vi "2012_12_14_local.vi"(0 "MC Power Data In":waveform(dbl)[](array[waveform]), 1 "Motor Power Data In":waveform(dbl)[](array[waveform]), 5 "Power \nSetting":i8(slide) min=0 max=100 step=10 scale=0.0..100.0, 7 "On/Off Control":T1(ring), 9 "Motor":i16=1, 11 "Error In":errorcluster, 12 "Fine Data In":dbl[][][](array[numeric])) -> (6 "Power \nSetting":i8(slide) min=0 max=100 step=10 scale=0.0..100.0, 14 "Fine Data Out":dbl[][][](array[numeric]), 15 "Errors":errorcluster)   [LabVIEW 2011]
uses:
  <vilib>/express/express arith-compare/Formula/XNode/ExpressFormulaBlockNode.xnode
  <vilib>/Analysis/NI_AALBase.lvlib
panel:
  in  "coarse path":path=path "Durability/coarse.lvm"
  in  "fine path":path=path "Durability/fine.lvm"
  out "Efficiency (%)":dbl format="%#.4f"
  in  "Manual Save\nFine Event":bool
  in  "Motor1 ID":string
  in  "User":string
  in  "Comments (cleared when written to file)":string
  out "Elapsed Time (s)":string caption="Elapsed Time Text"
  out "Start Time":string caption="Start Time Text"
  in  "Motor Failure\n(click to reset)":bool
  out "Coarse":bool caption="Time has Elapsed"
  out "Fine":bool caption="Time has Elapsed"
  out "Temps":dynamicdata(graph) caption="Signal Out"
  out "Power Graph":dynamicdata(graph) caption="Collected Signals"
  out "RPM":dynamicdata(graph) caption="Collected Signals"
  out "Motor RPM":dbl format="%#.0f"
  out "Power to Motor (W)":dbl format="%#.4f"
  out "Power to MC (W)":dbl format="%#.4f"
  out "Supply Voltage (V)":dbl format="%#.4f"
  in  "Record":bool
  out "Motor Temp (F)":dbl format="%.1f"
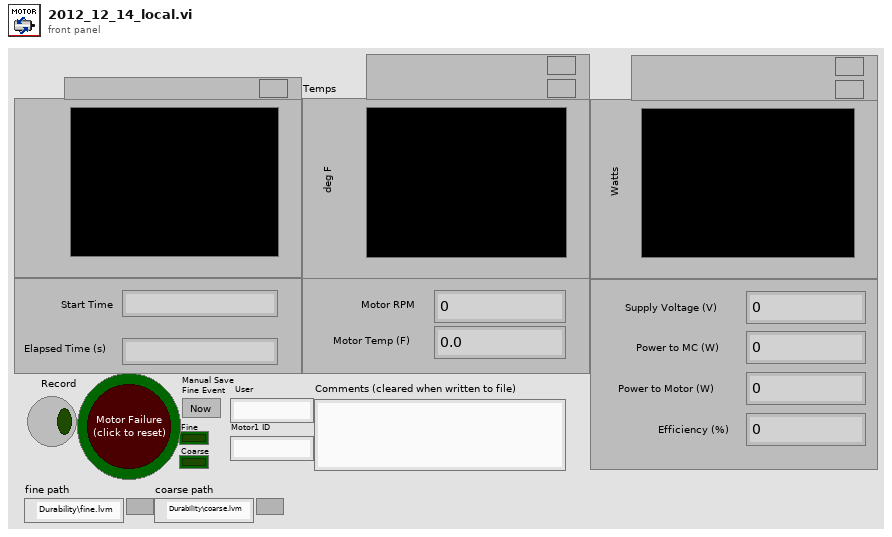
[diagram p1: front panel]
types:
  T1 = enum8{"Enabled", "Disabled", "Disabled and Grayed Out"}
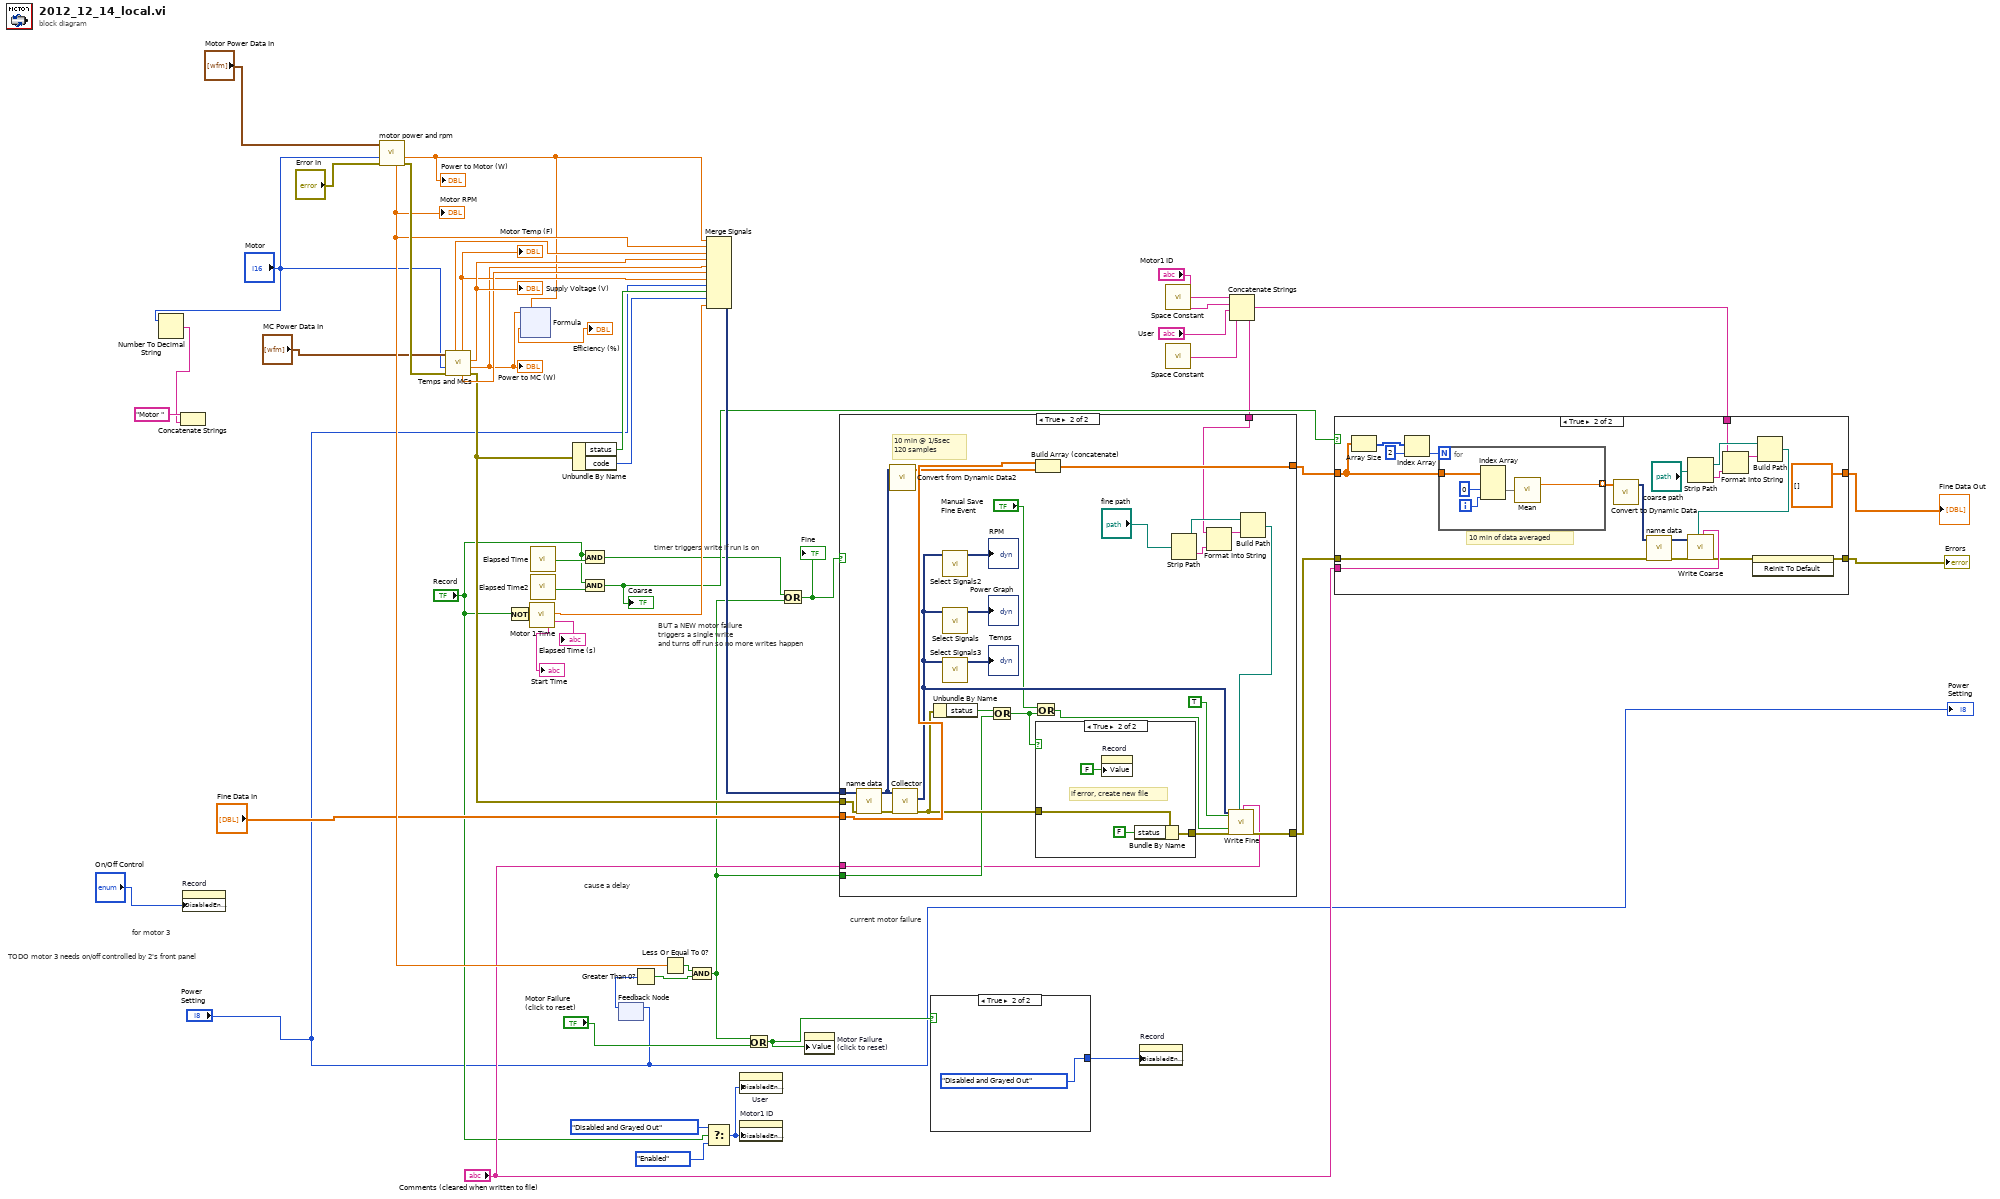
[diagram p0: block diagram]
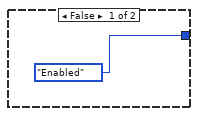
[diagram p2: hidden frame]
diagram:
  # "TODO motor 3 needs on/off controlled by 2's front panel"
  # "for motor 3"
  # "cause a delay"
  # "timer triggers write if run is on"
  # "BUT a NEW motor failure\ntriggers a single write\nand turns off run so no more writes happen"
  # "current motor failure"
  n1 = Number To Decimal String(number="Motor") -> (decimal integer string=w14:string)  [unwired: 1 in]
  n2 = Concatenate Strings("Motor ", w14) -> ()  [unwired: 1 out]
  n3 = property on="Record" class="Bool (strict)"("DisabledEnum"="On/Off Control") -> ()  [unwired: 2 in, 2 out]
  n4 = call "motor power and rpm.vi"("error in (no error)"="Error In", "Motor"="Motor", "data"="Motor Power Data In") -> ("error out"=w52:errorcluster, "Power"=w29:dbl, "RPM"=w42:dbl)  [unwired: 4 in, 2 out]
  "Motor RPM" <- w42
  "Power to Motor (W)" <- w29
  n5 = call "Temps and MCs.vi"("error in (no error)"=w52, "Motor"="Motor", "data"="MC Power Data In") -> ("error out"=w17:errorcluster, "Power 1"=w28:dbl, "Voltage 1"=w47:dbl, "Tank Temp"=w46:dbl, "Motor Temp"=w45:dbl, "Current 1"=w51:dbl)  [unwired: 3 in]
  "Motor Temp (F)" <- w45
  "Supply Voltage (V)" <- w47
  "Power to MC (W)" <- w28
  n6 = Not(x="Record") -> (.not. x?=w37:bool)
  n7 = xnode ("Formula")("MC PWR"=w28, "M PWR"=w29) -> ("Result"=→"Efficiency (%)":dbl)  [unwired: 1 in, 1 out]
  n8 = call "Motor 1 Time"("Reset"=w37) -> ("Start Time Text"=→"Start Time":string, "Elapsed Time (s)"=w36:dbl, "Elapsed Time Text"=→"Elapsed Time (s)":string)  [unwired: 11 in, 5 out]
  n9 = call "Elapsed Time"() -> ("Time has Elapsed"=w30:bool)  [unwired: 12 in, 7 out]
  n10 = call "Elapsed Time2"() -> ("Time has Elapsed"=w32:bool)  [unwired: 12 in, 7 out]
  n11 = Unbundle By Name(w17) -> ("status"=w50:bool, "code"=w49:i32)
  n12 = And(x="Record", y=w30) -> (x .and. y?=w5:bool)
  n13 = And(x="Record", y=w32) -> (x .and. y?=w31:bool)
  "Coarse" <- w31
  n14 = feedback-in #1("Power \nSetting") -> ()
  n15 = feedback #1() -> (w6:i8)  [unwired: 1 in]
  n16 = Greater Than 0?(x=w6) -> (x > 0?=w40:bool)
  n17 = Less Or Equal To 0?(x=w42) -> (x <= 0?=w41:bool)
  n18 = And(x=w41, y=w40) -> (x .and. y?=w4:bool)
  n19 = Merge Signals(w29, w42, w51, w47, w28, w46, w45, "Power \nSetting", w50, w49, w36) -> (w48:dynamicdata)
  n20 = Select(t=T1."Disabled and Grayed Out" ("Disabled"), s="Record", f=T1."Enabled" ("Disabled")) -> (s? t:f=w33:T1)
  n21 = property on="User" class="Str"("DisabledEnum"=w33) -> ()  [unwired: 2 in, 2 out]
  n22 = property on="Motor1 ID" class="Str"("DisabledEnum"=w33) -> ()  [unwired: 2 in, 2 out]
  n23 = Or(x=w4, y="Motor Failure\n(click to reset)") -> (x .or. y?=w2:bool)
  n24 = Or(x=w5, y=w4) -> (x .or. y?=w7:bool)
  "Fine" <- w7
  n25 = property on="Motor Failure\n(click to reset)" class="Bool (strict)"("Value"=w2) -> ()  [unwired: 2 in, 2 out]
  n26 = case shown="True" w2 {
    tunnel: [T1."Enabled" ("Disabled") T1."Disabled and Grayed Out" ("Disabled")] -> w9
    frame False {
    }
    frame True {
    }
  }
  n27 = property on="Record" class="Bool (strict)"("DisabledEnum"=w9) -> ()  [unwired: 2 in, 2 out]
  n28 = call <vilib>:"Space Constant.vi"() -> ("String"=w23:string)
  n29 = call <vilib>:"Space Constant.vi"() -> ("String"=w21:string)
  n30 = Concatenate Strings("Motor1 ID", w23, "User", w21) -> (w20:string)
  n31 = case shown="True" w7 {
    tunnel: w48 -> [_ w79]
    tunnel: w17 -> [w56 w76]
    tunnel: [w56 w71] -> w8
    tunnel: [w55 w83] -> w43
    tunnel: "Fine Data In" -> [w55 w82]
    tunnel: w4 -> [_ w68]
    tunnel: "Comments (cleared when written to file)" -> [_ w67]
    tunnel: w20 -> [_ w60]
    frame False {
    }
    frame True {
      # "10 min @ 1/5sec\n120 samples"
      n32 = call "name data.vi"("error in (no error)"=w76, "Dynamic Data"=w79) -> ("error out"=w77:errorcluster, "Output"=w78:dynamicdata)  [unwired: 8 in]
      n33 = call "Convert from Dynamic Data2"("Dynamic Data Type"=w78) -> ("Array"=w81:dbl[][])  [unwired: 3 in]
      n34 = call "Collector"("error in (no error)"=w77, "Signals"=w78) -> ("error out"=w69:errorcluster, "Collected Signals"=w72:dynamicdata)  [unwired: 8 in]
      n35 = Unbundle By Name(w69) -> ("status"=w58:bool)
      n36 = call "Select Signals2"("Signals"=w72) -> ("Signal Out"=→"RPM":dynamicdata)  [unwired: 9 in, 1 out]
      n37 = call "Select Signals"("Signals"=w72) -> ("Signal Out"=→"Power Graph":dynamicdata)  [unwired: 9 in, 1 out]
      n38 = call "Select Signals3"("Signals"=w72) -> ("Signal Out"=→"Temps":dynamicdata)  [unwired: 9 in, 1 out]
      n39 = Or(x=w58, y=w68) -> (x .or. y?=w57:bool)
      n40 = Or(x="Manual Save\nFine Event", y=w57) -> (x .or. y?=w66:bool)
      n41 = Build Array (concatenate)(w82, w81) -> (w83:dbl[][][])
      n42 = case shown="True" w57 {
        tunnel: [w84 w88] -> w70
        tunnel: w69 -> [w84 w87]
        frame False {
        }
        frame True {
          # "if error, create new file"
          n43 = property on="Record" class="Bool (strict)"("Value"=FALSE ("Manual Start")) -> ()  [unwired: 2 in, 2 out]
          n44 = Bundle By Name(cluster=w87, "status"=FALSE) -> (w88:errorcluster)
        }
      }
      n45 = Strip Path(path="fine path") -> (stripped path=w63:path, name=w59:string)
      n46 = Format Into String(initial string=w60, w59) -> (resulting string=w64:string)  [unwired: 2 in, 1 out]
      n47 = Build Path(base path=w63, name or relative path=w64) -> (appended path=w61:path)
      n48 = call "Write Fine"("Signals"=w72, "Reset"=TRUE, "new_file"=w66, "error in (no error)"=w70, "Filename"=w61, "Comment"=w67) -> ("error out"=w71:errorcluster)  [unwired: 11 in, 2 out]
    }
  }
  n49 = case shown="True" w31 {
    tunnel: w43 -> [w90 w109]
    tunnel: [w90 dbl[][][] []] -> w44
    tunnel: w8 -> [w89 w101]
    tunnel: [w89 w97] -> w26
    tunnel: "Comments (cleared when written to file)" -> [_ w99]
    tunnel: w20 -> [_ w92]
    frame False {
    }
    frame True {
      # "10 min of data averaged"
      n50 = Array Size(array=w109) -> (size(s)=w105:i32[])
      n51 = Index Array(array=w105, index=2) -> (element=w106:i32)
      n52 = for {
        N: w106 -> [_]
        tunnel: w109 -> [w114]
        tunnel: [w110] -> w104 mode=indexing
        i -> [w113]
        n53 = Index Array(array=w114, index (dim 1)=0 ("disabled index (row)"), index (dim 2)=w113) -> (element=w112:dbl[])  [unwired: 1 in]
        n54 = call <vilib>:"Mean.vi"("X"=w112) -> ("mean"=w110:dbl)  [unwired: 1 out]
      }
      n55 = call "Convert to Dynamic Data"("Array"=w104) -> ("Dynamic Data Type"=w103:dynamicdata)  [unwired: 3 in]
      n56 = call "name data.vi"("error in (no error)"=w101, "Dynamic Data"=w103) -> ("error out"=w100:errorcluster, "Output"=w102:dynamicdata)  [unwired: 8 in]
      n57 = Strip Path(path="coarse path") -> (stripped path=w95:path, name=w93:string)
      n58 = Format Into String(initial string=w92, w93) -> (resulting string=w94:string)  [unwired: 2 in, 1 out]
      n59 = Build Path(base path=w95, name or relative path=w94) -> (appended path=w91:path)
      n60 = call "Write Coarse"("Signals"=w102, "error in (no error)"=w100, "Filename"=w91, "Comment"=w99) -> ("error out"=w98:errorcluster)  [unwired: 13 in, 2 out]
      n61 = invoke on="Comments (cleared when written to file)" class="Str" method="Reinit To Default"(error in=w98) -> (error out=w97:errorcluster)  [unwired: 2 in, 2 out]
    }
  }
  "Errors" <- w26
  "Fine Data Out" <- w44
  "Power \nSetting" <- "Power \nSetting"
